vi "Variable Common Setup GUI.vi"(11 "error in (no error)":errorcluster) -> (8 "OK":bool, 15 "error out":errorcluster)   [LabVIEW 2011]
uses:
  User Setting Analog Channel Bg.ctl
  Scaling.ctl
  Alarm Setup Analog.ctl
  Alarm Responce.ctl
  Action List.ctl
  Limits.ctl
  Update frequensies.ctl
  Common/Variable List Common Analog.ctl
  <vilib>/Utility/VariantDataType/GetNumericInfo.vi
panel:
  out "Sampling Rate":T1
  out "Description":string
  out "Unit":string
  out "Name":string
  in  "User Selectable":T2 {"Scaling"."Offset" format="%.5f"; "Scaling"."Gain" format="%.5f"; "Limits and responces"."Limits"."H" format="%.3f"; "Limits and responces"."Limits"."L" format="%.3f"; "Limits and responces"."Limits"."HH" format="%.3f"; "Limits and responces"."Limits"."LL" format="%.3f"; "Limits and responces"."HH"."Action" items=["No Action", "Turn Off HV"]; "Limits and responces"."H"."Action" items=["No Action", "Turn Off HV"]; "Limits and responces"."L"."Action" items=["No Action", "Turn Off HV"]; "Limits and responces"."LL"."Action" items=["No Action", "Turn Off HV"]; "Limits and responces"."Technical Error(NA)"."Action" items=["No Action", "Turn Off HV"]}
  in  "List of variables":i32(listbox)
  out "Mode":bool
  in  "Help":bool
  in  "Cancel":bool
  in  "OK btn":bool
  # "Information"
  # "Tab header s can be changed as wanted\n\nCustom can be used for completly ccutom behavior,\nmust then highjack  an other hidden page, for settings"
  # "Add custom behavior taht cvan not be replicated by a simple cluster with valisdity checking"
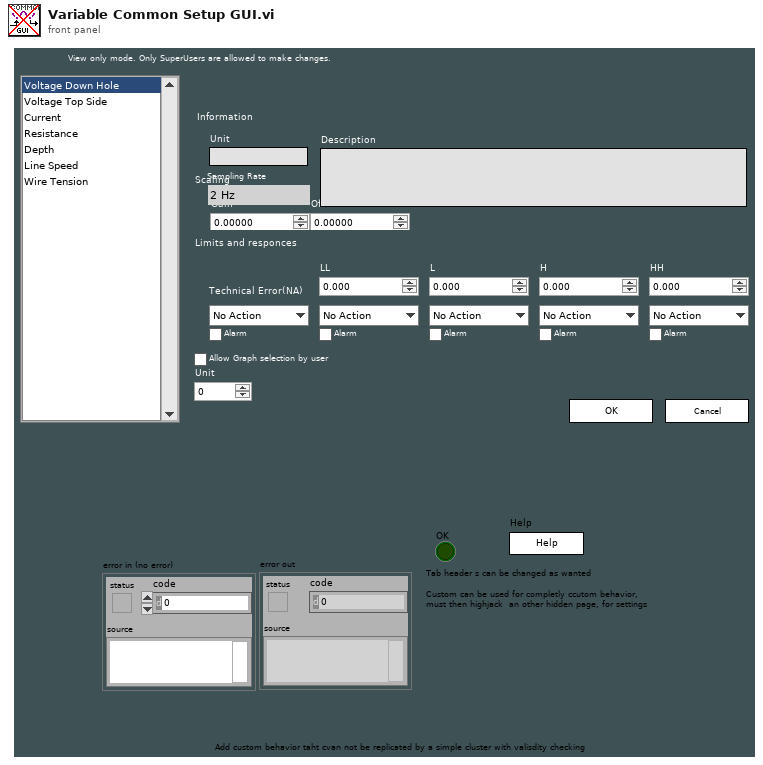
[diagram p1: front panel]
types:
  T1 = typedef "Update frequensies.ctl" = enum16{"2 Hz", "1 Hz", "0.1 Hz"}
  T2 = typedef "User Setting Analog Channel Bg.ctl" = cluster{"Scaling":T3, "Limits and responces":T4, "Allow Graph selection by user":bool, "Unit":u16}
  T3 = typedef "Scaling.ctl" = cluster{"Gain":dbl, "Offset":dbl}
  T4 = typedef "Alarm Setup Analog.ctl" = cluster{"Technical Error(NA)":T5, "LL":T5, "L":T5, "H":T5, "HH":T5, "Limits":T7}
  T5 = typedef "Alarm Responce.ctl" = cluster{"Action":T6, "Alarm":bool}
  T6 = typedef "Action List.ctl" = u16
  T7 = typedef "Limits.ctl" = cluster{"LL":dbl, "L":dbl, "H":dbl, "HH":dbl}
  T8 = enum16{"GET", "SET", "Get from Ini", "Put in Ini"}
  T9 = typedef "User Indikator.ctl" = cluster{"User Name":string, "Super User":T10}
  T10 = typedef "Super User bool indikator.ctl" = bool
  T11 = typedef "Variable List Common Analog.ctl" = enum16{"HVPSU Head Voltage", "HVPSU TS Voltage", "HVPSU Current", "PCP Cable Resistance", "Winch Depth", "Winch Line Speed", "Winch Wire Tension"}
  T12 = enum8{"Enabled", "Disabled", "Disabled and Grayed Out"}
  T13 = typedef "Fixed Analog Channel Definition.ctl" = cluster{"ID":u16, "Name":string, "Quantity":T14, "Unit":string, "Maximum upd":T1, "Comment":string, "Help file Name":string, "Help file Section ":string, "Category":T15, "User adjustable Scaling":bool, "Default Scaling":T3, "In use":bool, "Default Unit":i32}
  T14 = typedef "Quantity enum.ctl" = enum16{"Acceleration", "Angle", "Current", "Force", "Distance", "Pressure", "Resistance", "Rotational Speed", "Speed", "Temperature", "Tension", "Torque", "Voltage", "Weight"}
  T15 = typedef "Channel catagory Enum.ctl" = enum16{"No Category", "Power", "Temperature", "Pressure"}
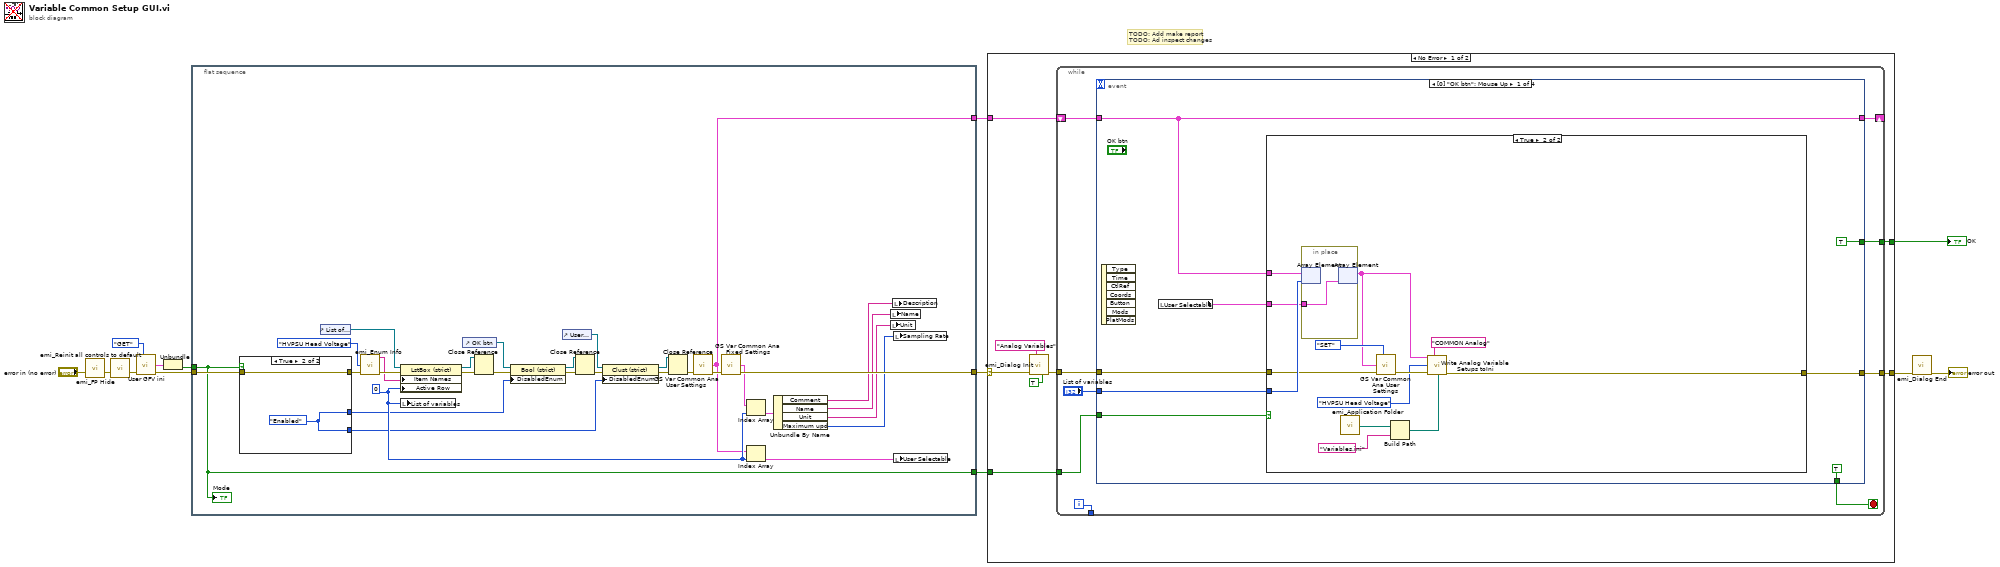
[diagram p0: block diagram]
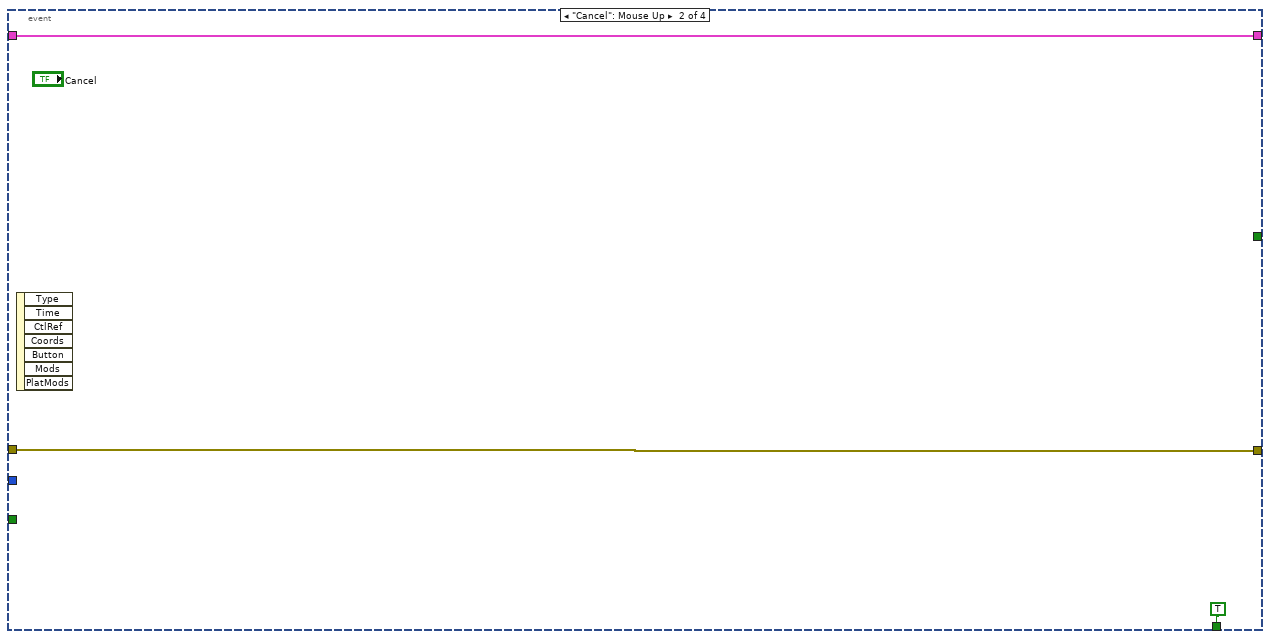
[diagram p3: hidden frame]
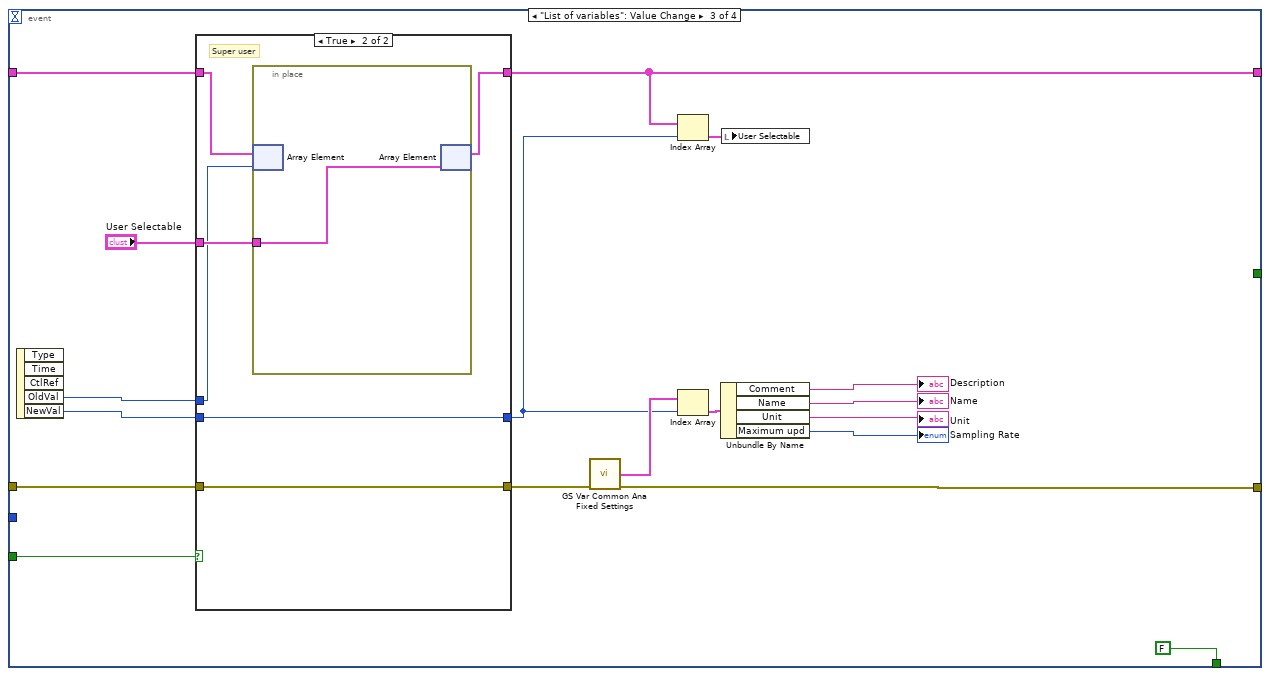
[diagram p4: hidden frame]
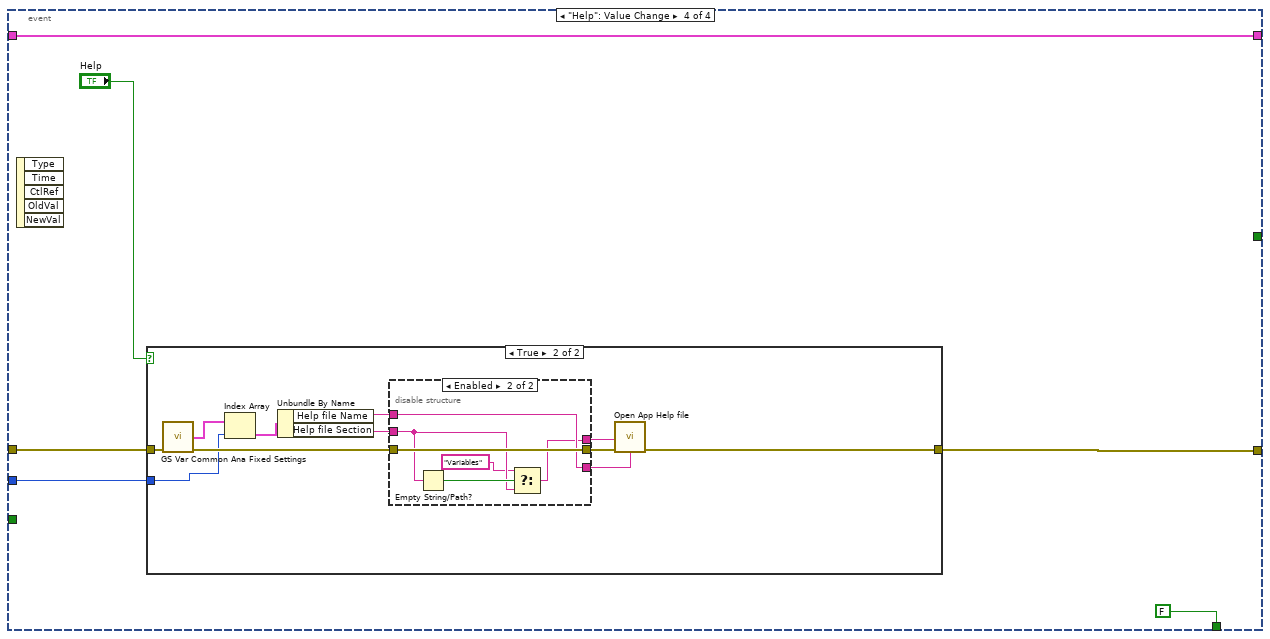
[diagram p6: hidden frame]
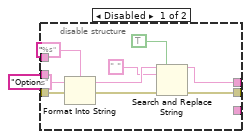
[diagram p8: hidden frame]
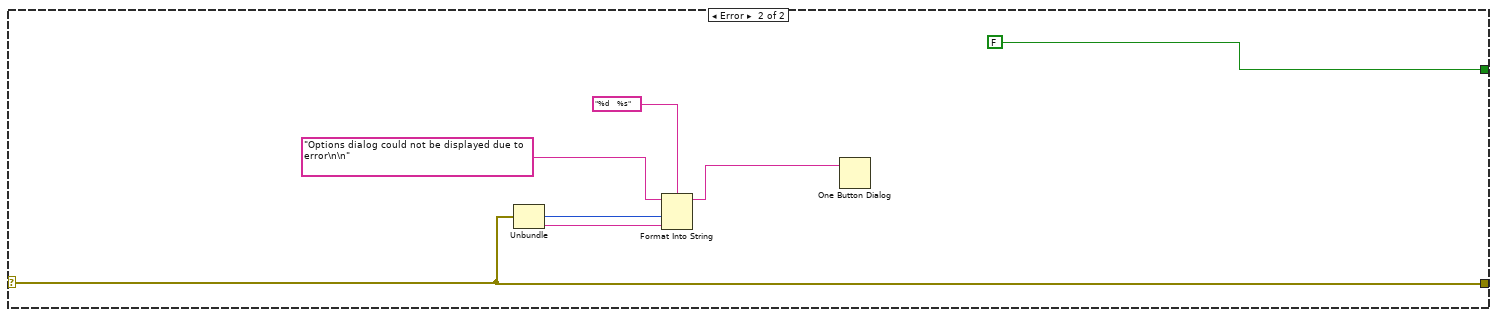
[diagram p9: hidden frame]
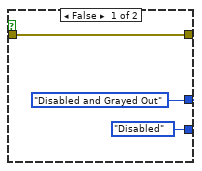
[diagram p10: hidden frame]
diagram:
  # "TODO: Add make report\nTODO: Ad inspect changes"
  n1 = call "emi_FP Hide.vi"("error in (no error)"="error in (no error)") -> ("error out"=w9:errorcluster)  [unwired: 13 in, 1 out]
  n2 = call "emi_Reinit all controls to default.vi"("error in (no error)"=w9) -> ("error out"=w7:errorcluster)  [unwired: 13 in, 1 out]
  n3 = call "User GFV ini.vi"("Action(GET)"=T8."GET", "error in (no error)"=w7) -> ("User ID out"=w6:T9, "error out"=w5:errorcluster)  [unwired: 12 in]
  n4 = Unbundle(w6) -> ("Super User"=w4:T10)  [unwired: 1 out]
  n5 = flat-sequence {
    tunnel: [w31] -> w8
    tunnel: w5 -> [w44]
    tunnel: w4 -> [w17]
    tunnel: [w17] -> w3
    tunnel: [w16] -> w2
    frame #0 {
      w30 = 0 ("Active Row:Active Row Number")
      n6 = case shown="True" w17 {
        tunnel: w44 -> [w46 w49]
        tunnel: [w46 w49] -> w40
        tunnel: [T12."Disabled and Grayed Out" ("Disabled") w48] -> w14
        tunnel: [T12."Disabled" ("Disabled") w48] -> w15
        frame False {
        }
        frame True {
          w48 = T12."Enabled" ("Disabled")
        }
      }
      n7 = control-ref of="List of variables"() -> (w37:refnum<vi>)
      n8 = call "emi_Enum Info.vi"("Enum"=Variable_List_Common_Analog."HVPSU Head Voltage" ("Action"), "error in (no error)"=w40) -> ("Text Elements"=w33:string[], "error out"=w38:errorcluster)  [unwired: 10 in, 2 out]
      n9 = property class="LstBox (strict)"(reference=w37, error in=w38, "Item Names"=w33, "Active Row"=w30) -> (reference out=w35:refnum<vi>, error out=w36:errorcluster)
      n10 = local write "List of variables"(w30) -> ()
      n11 = control-ref of="OK btn"() -> (w43:refnum<vi>)
      n12 = Close Reference(reference=w35, error in (no error)=w36) -> (error out=w34:errorcluster)
      n13 = property class="Bool (strict)"(reference=w43, error in=w34, "DisabledEnum"=w14) -> (reference out=w41:refnum<vi>, error out=w42:errorcluster)
      n14 = control-ref of="User Selectable"() -> (w18:refnum<vi>)
      n15 = Close Reference(reference=w41, error in (no error)=w42) -> (error out=w19:errorcluster)
      n16 = property class="Clust (strict)"(reference=w18, error in=w19, "DisabledEnum"=w15) -> (reference out=w22:refnum<vi>, error out=w21:errorcluster)
      n17 = Close Reference(reference=w22, error in (no error)=w21) -> (error out=w20:errorcluster)
      n18 = call "GS Var Common Ana User Settings.vi"("error in (no error)"=w20) -> ("Common Analog var User set out"=w16:T2[], "error out"=w32:errorcluster)  [unwired: 12 in, 1 out]
      n19 = call "GS Var Common Ana Fixed Settings.vi"("error in (no error)"=w32) -> ("Common Analog Var Fixed out"=w29:T13[], "error out"=w31:errorcluster)  [unwired: 12 in, 1 out]
      n20 = Index Array(array=w29, index=w30) -> (element=w28:T13)
      n21 = Index Array(array=w16, index=w30) -> (element=w23:T2)
      n22 = Unbundle By Name(w28) -> ("Comment"=w24:string, "Name"=w25:string, "Unit"=w26:string, "Maximum upd"=w27:T1)
      n23 = local write "Unit"(w26) -> ()
      n24 = local write "Name"(w25) -> ()
      n25 = local write "Description"(w24) -> ()
      n26 = local write "Sampling Rate"(w27) -> ()
      n27 = local write "User Selectable"(w23) -> ()
      "Mode" <- w17
    }
  }
  n28 = case shown="No Error" w8 {
    selector: w8 -> [w52 w159]
    tunnel: [w57 FALSE] -> w12
    tunnel: [w56 w159] -> w11
    tunnel: w3 -> [w51 _]
    tunnel: w2 -> [w50 _]
    frame No Error {
      n29 = call "emi_Dialog Init.vi"("Header String(\"\")"="Analog Variables" ("Header String(\"\")"), "error in"=w52, "Modal(T)"=TRUE) -> ("error out"=w55:errorcluster)  [unwired: 12 in]
      n30 = while {
        tunnel: [w66] -> _
        tunnel: w55 -> [w64]
        tunnel: [w63] -> w56
        tunnel: [w62] -> w57
        tunnel: w51 -> [w61]
        shift-right: [w59] -> _
        shift-left: w50 -> [w60]
        i -> [w66]
        stop <- w65 stop-if-true
        n31 = event shown="[0] \"OK btn\": Mouse Up" {
          selector: _ -> [_ _ _ _]
          dyn-events: _ -> [_ _ _ _]
          timeout: _ -> [_ _ _ _]
          tunnel: [TRUE TRUE FALSE FALSE] -> w65
          tunnel: w64 -> [w73 w91 w108 w124]
          tunnel: [w72 w91 w101 w125] -> w63
          tunnel: [TRUE _ _ _] -> w62
          tunnel: w61 -> [w71 _ w109 _]
          tunnel: w60 -> [w70 w90 w107 w122]
          tunnel: [w70 w90 w95 w122] -> w59
          tunnel: "List of variables" -> [w69 _ _ w121]
          event "OK btn": Mouse Up {
            n32 = event-data() -> ()  [unwired: 1 in, 7 out]
            n33 = local read "User Selectable"() -> (w68:T2)
            n34 = case shown="True" w71 {
              tunnel: w73 -> [w75 w85]
              tunnel: [w75 w80] -> w72
              tunnel: w70 -> [_ w88]
              tunnel: w69 -> [_ w87]
              tunnel: w68 -> [_ w86]
              frame False {
              }
              frame True {
                n35 = in-place {
                  in-place-border: w86 -> [w89]
                  n36 = in-place-array #1(w88, w87) -> ()  [unwired: 1 out]
                  n37 = in-place-array #1(w89) -> (w81:T2[])  [unwired: 1 out]
                }
                n38 = call "emi_Application Folder.vi"() -> ("Dir"=w78:path)  [unwired: 14 in, 1 out]
                n39 = call "GS Var Common Ana User Settings.vi"("Action(GET)"=enum16{"GET", "SET"}."SET", "Common variables User settigns in"=w81, "error in (no error)"=w85) -> ("error out"=w83:errorcluster)  [unwired: 10 in, 2 out]
                n40 = Build Path(base path=w78, name or relative path="Variables.ini") -> (appended path=w76:path)
                n41 = call "Write Analog Variable Setups toIni.vi"("error in (no error)"=w83, "Path"=w76, "Enum with Variable List"=Variable_List_Common_Analog."HVPSU Head Voltage" ("Action"), "Analog User settigns"=w81, "Section(\"Default\")"="COMMON Analog" ("Section(\"Default\")")) -> ("error out"=w80:errorcluster)  [unwired: 10 in]
              }
            }
          }
          event "Cancel": Mouse Up {
            n42 = event-data() -> ()  [unwired: 1 in, 7 out]
          }
          event "List of variables": Value Change {
            n43 = event-data() -> ("OldVal"=w106:i32, "NewVal"=w105:i32)  [unwired: 1 in, 3 out]
            n44 = case shown="True" w109 {
              tunnel: [w111 w119] -> w102
              tunnel: w108 -> [w111 w119]
              tunnel: w107 -> [w113 w118]
              tunnel: [w113 w117] -> w95
              tunnel: "User Selectable" -> [_ w116]
              tunnel: w106 -> [_ w115]
              tunnel: w105 -> [w112 w114]
              tunnel: [w112 w114] -> w94
              frame False {
              }
              frame True {
                # "Super user"
                n45 = in-place {
                  in-place-border: w116 -> [w120]
                  n46 = in-place-array #2(w118, w115) -> ()  [unwired: 1 out]
                  n47 = in-place-array #2(w120) -> (w117:T2[])  [unwired: 1 out]
                }
              }
            }
            n48 = call "GS Var Common Ana Fixed Settings.vi"("error in (no error)"=w102) -> ("Common Analog Var Fixed out"=w104:T13[], "error out"=w101:errorcluster)  [unwired: 12 in, 1 out]
            n49 = Index Array(array=w95, index=w94) -> (element=w93:T2)
            n50 = Index Array(array=w104, index=w94) -> (element=w103:T13)
            n51 = Unbundle By Name(w103) -> ("Comment"=→"Description":string, "Name"=→"Name":string, "Unit"=→"Unit":string, "Maximum upd"=→"Sampling Rate":T1)
            n52 = local write "User Selectable"(w93) -> ()
          }
          event "Help": Value Change {
            n53 = event-data() -> ()  [unwired: 1 in, 5 out]
            n54 = case shown="True" "Help" {
              tunnel: [w127 w138] -> w125
              tunnel: w124 -> [w127 w135]
              tunnel: w121 -> [_ w128]
              frame False {
              }
              frame True {
                n55 = call "GS Var Common Ana Fixed Settings.vi"("error in (no error)"=w135) -> ("Common Analog Var Fixed out"=w132:T13[], "error out"=w134:errorcluster)  [unwired: 12 in, 1 out]
                n56 = Index Array(array=w132, index=w128) -> (element=w133:T13)
                n57 = Unbundle By Name(w133) -> ("Help file Name"=w130:string, "Help file Section"=w129:string)
                n58 = disable-structure shown="Enabled" {
                  disable-tunnel: w134 -> [w147 w153]
                  disable-tunnel: [w143 w153] -> w137
                  disable-tunnel: [w139 w149] -> w136
                  disable-tunnel: [_ w152] -> w131
                  disable-tunnel: w130 -> [_ w152]
                  disable-tunnel: w129 -> [_ w150]
                  frame Disabled {
                    n59 = Format Into String(format string="%s", initial string="Options", error in=w147) -> (resulting string=w141:string, error out=w144:errorcluster)  [unwired: 1 in]
                    n60 = Search and Replace String(replace all?=TRUE ("replace all? (F)"), input string=w141, search string=" ", error in=w144) -> (result string=w139:string, error out=w143:errorcluster)  [unwired: 4 in, 2 out]
                  }
                  frame Enabled {
                    n61 = Empty String/Path?(string/path=w150) -> (empty?=w151:bool)
                    n62 = Select(t="Variables", s=w151, f=w150) -> (s? t:f=w149:string)
                  }
                }
                n63 = call "Open App Help file.vi"("Help Tag (\"\")"=w136, "error In"=w137, "file name(\"App\".chm)"=w131) -> ("error out"=w138:errorcluster)  [unwired: 12 in]
              }
            }
          }
        }
      }
    }
    frame Error {
      n64 = Unbundle(w159) -> ("code"=w156:i32, "source"=w155:string)  [unwired: 1 out]
      n65 = Format Into String(format string="%d    %s", initial string="Options dialog could not be displayed due to error\n\n" ("message"), w156, w155) -> (resulting string=w157:string)  [unwired: 1 in, 1 out]
      n66 = One Button Dialog(message=w157) -> ()  [unwired: 1 in, 1 out]
    }
  }
  "OK" <- w12
  n67 = call "emi_Dialog End.vi"("error in"=w11) -> ("error out"=→"error out":errorcluster)  [unwired: 14 in]
